vi "TransmissionShift.vi"(0 "Value":T1, 4 "Synchronization":enum16{"Start", "Wait"}(ring)) -> (10 "Command Info Out":T2)   [LabVIEW 2019]
doc: "This template has a parameter to control whether it waits for the command to complete or not. This is useful for operations that have a timed duration or a sensor-based duration. \n\nBe sure to right-click and select New from Template and save with a new command name."
uses:
  <vilib>/Rock Robotics/WPI/Framework/Command Status Info.ctl
  <vilib>/Rock Robotics/WPI/Framework/Completion Status.ctl
  <vilib>/Rock Robotics/WPI/Framework/Completion Notifier.ctl
  <vilib>/Rock Robotics/WPI/Solenoid/WPI_SolenoidValue.ctl
  Implementation/Pnuematics Setpoints.ctl
  Implementation/Pnuematics Operations.ctl
panel:
  in  "Command Info In":T2
  in  "Description":string
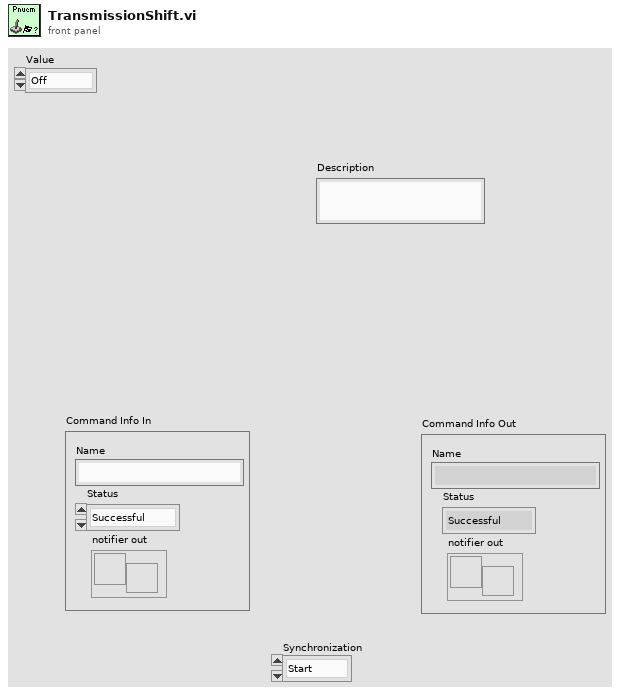
[diagram p1: front panel]
types:
  T1 = typedef "WPI_SolenoidValue.ctl" = enum16{"Off", "On", "Forward", "Reverse"}
  T2 = typedef "Command Status Info.ctl" = cluster{"Name":string, "Status":T3, "notifier out":T4}
  T3 = typedef "Completion Status.ctl" = enum16{"Successful", "Aborted", "Incomplete"}
  T4 = typedef "Completion Notifier.ctl" = refnum<notifier>
  T5 = typedef "Pnuematics Setpoints.ctl" = cluster{"Operation":T6, "Value":T1, "Solenoid":enum16{"Transmission", "Wheel"}, "Milliseconds":dbl}
  T6 = typedef "Pnuematics Operations.ctl" = enum16{"Reserve", "Read Current", "CompressorStart", "CompressorStop", "Solenoid", "TimedSolenoid", "Immediate"}
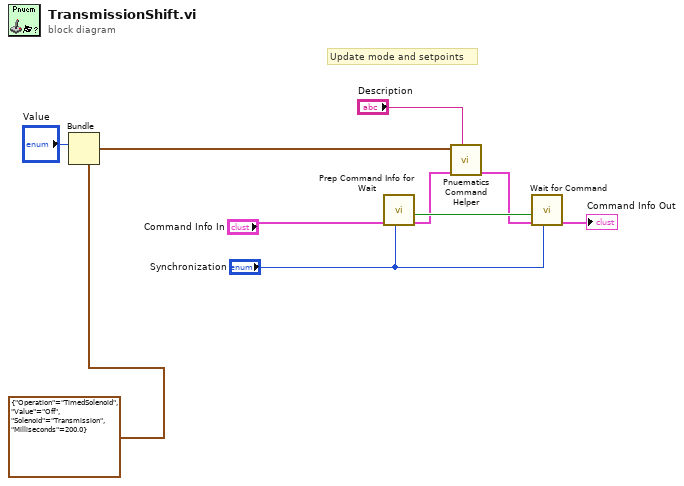
[diagram p0: block diagram]
diagram:
  # "Update mode and setpoints"
  n1 = Bundle(cluster=T5 {"Operation"=enum."TimedSolenoid", "Value"=enum."Off", "Solenoid"=enum."Transmission", "Milliseconds"=200.0} ("SubSystem Data"), "Value"="Value") -> (w3:T5)  [unwired: 3 in]
  n2 = call <vilib>:"Prep Command Info for Wait.vi"("Synchronication"="Synchronization", "Command Info"="Command Info In") -> ("Command Info"=w8:T2, "Allocated"=w9:bool)  [unwired: 8 in]
  n3 = call "Pnuematics Command Helper.vi"("Description"="Description", "Command Info In"=w8, "SubSystem Data"=w3) -> ("Command Info Out"=w5:T2)  [unwired: 6 in, 2 out]
  n4 = call <vilib>:"Wait for Command.vi"("Synchronication"="Synchronization", "Command Info in"=w5, "Allocated"=w9) -> ("Command Info out"=→"Command Info Out":T2)  [unwired: 8 in]
